vi "VI Server_Set Control Values from String Formats.vi"(6 "Options":T1, 8 "error in (no error)":errorcluster, 9 "Values":string[](array[string]), 10 "Labels":string[](array[string]), 11 "VI Server Cluster":T2={"Labels"=["Label", "Size", "Font", "Heght", "Width", "Ledding Denominator", "Ledding Nominator", "Label Number", "Microstep Resolution", "X", "Y", "Z", "Italic?", "Underlined?"], "Refs"=[], "VI Ref"=refnum}) -> (0 "error out":errorcluster, 3 "VI Server Cluster.DUP":T2={"Labels"=["Label", "Size", "Font", "Heght", "Width", "Ledding Denominator", "Ledding Nominator", "Label Number", "Microstep Resolution", "X", "Y", "Z", "Italic?", "Underlined?"], "Refs"=[], "VI Ref"=refnum}, 5 "FailedLabel":string)   [LabVIEW 2020, in "VI Server Toolkit LV2013.lvlib"]
doc: "<B>Set Control Values From String Formats.vi</B> and converts string values of the selected GUI objects onto original data type."
uses:
  VI Server Toolkit LV2013.lvlib
  VI Server_TypeDefs/VI Server_RefsCluster.ctl
  VI Server Libraries/VI Server Controls.llb/VI Server_GetSet Controls From String Format_Options.ctl
  <vilib>/userDefined/High Color/IMAQdx.ctl
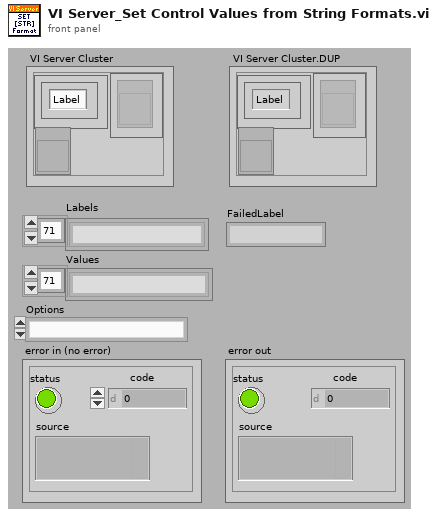
[diagram p1: front panel]
types:
  T1 = typedef "VI Server Toolkit LV2013.lvlib/VI Server_GetSet Controls From String Format_Options.ctl" = enum16{"", "If Ring Get Selection", "If Ring Set by Selection"}
  T2 = typedef "VI Server_RefsCluster.ctl" = cluster{"Labels":string[], "Refs":refnum<vi>[], "VI Ref":refnum<vi>}
  T3 = typedef "IMAQdx.ctl" = refnum<k21>
  T4 = typedef "LVStringsAndValuesArrayTypeDef_U32.ctl" = cluster{"String":string, "Value":u32}[]
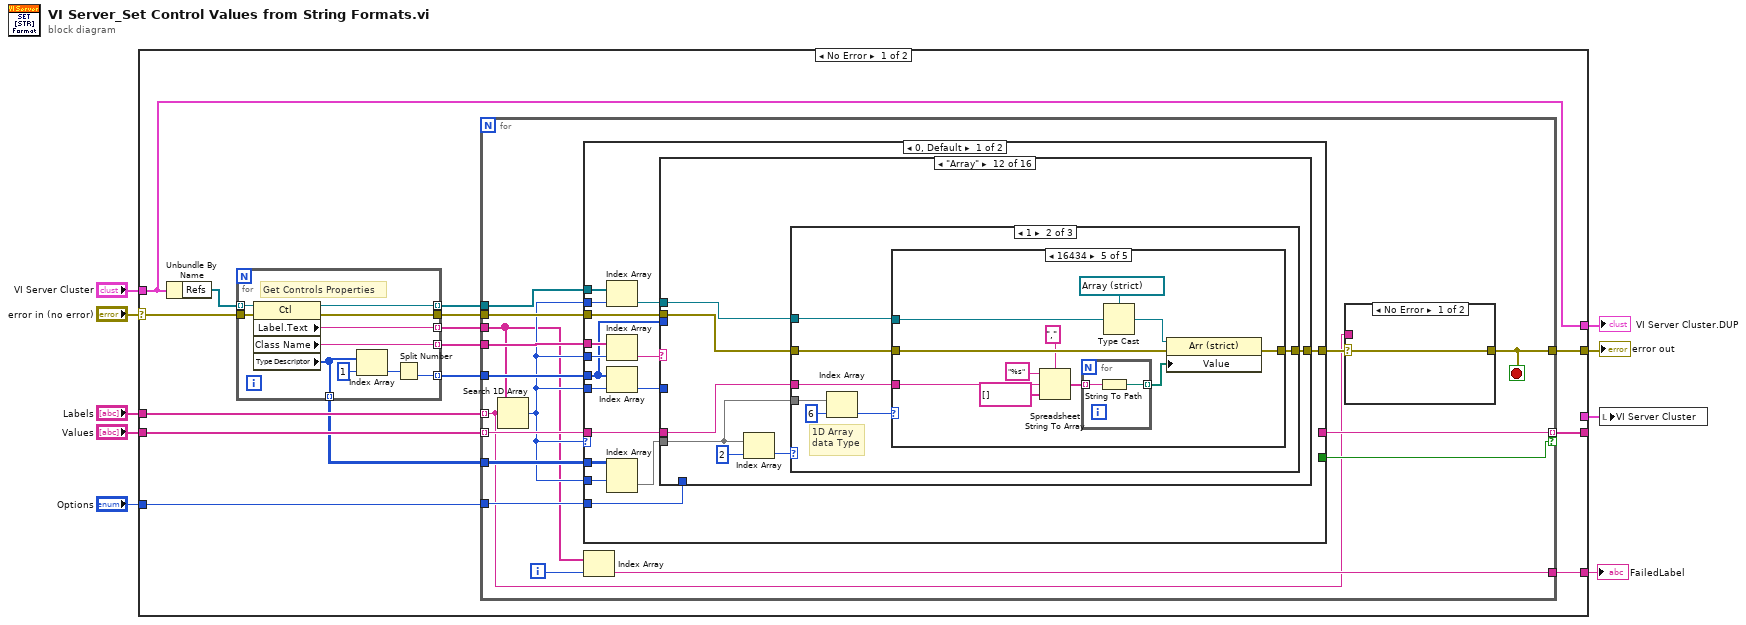
[diagram p0: block diagram]
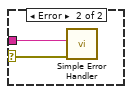
[diagram p2: hidden frame]
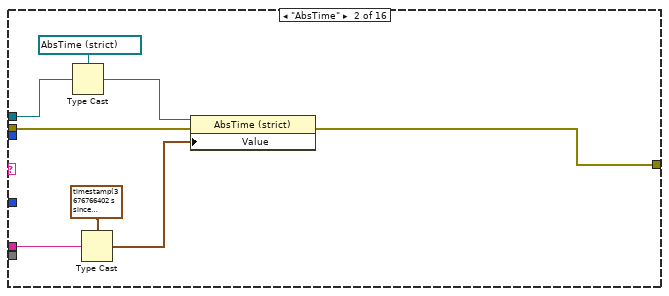
[diagram p4: hidden frame]
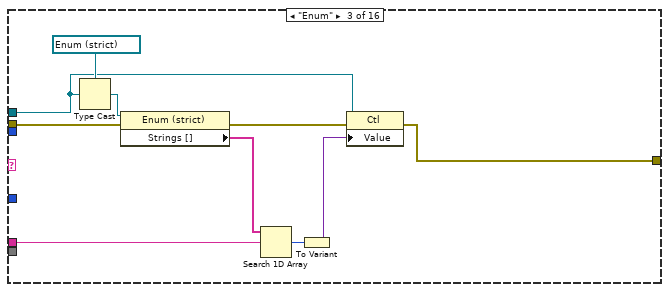
[diagram p5: hidden frame]
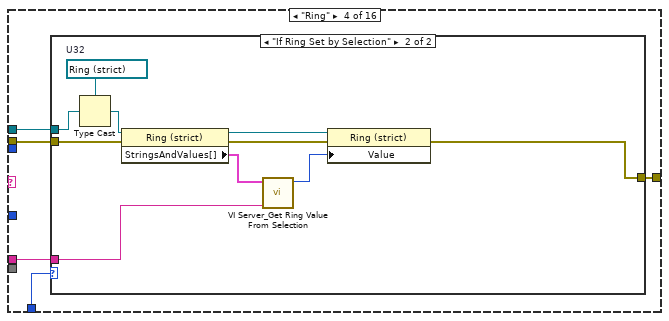
[diagram p6: hidden frame]
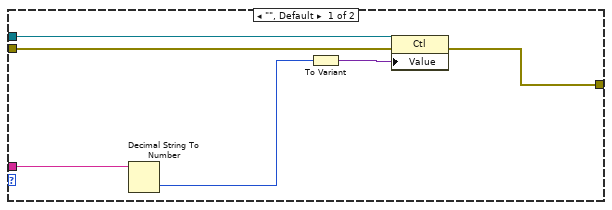
[diagram p7: hidden frame]
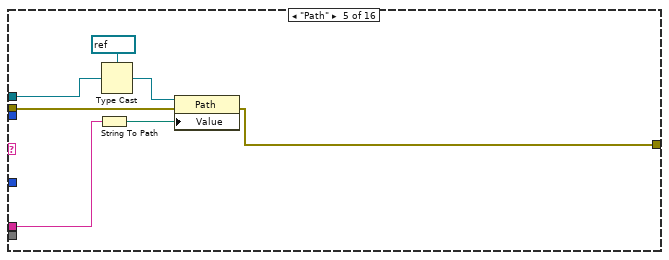
[diagram p8: hidden frame]
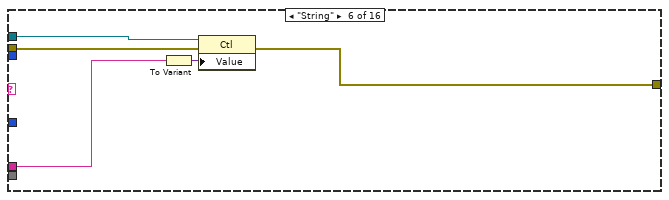
[diagram p9: hidden frame]
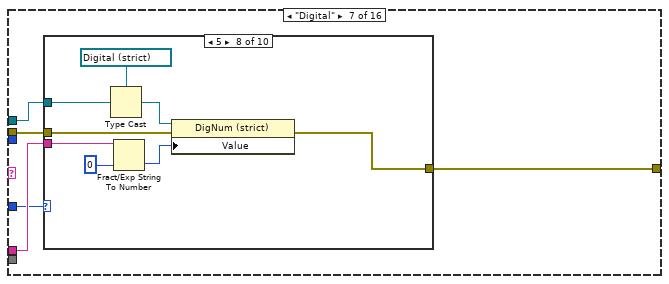
[diagram p10: hidden frame]
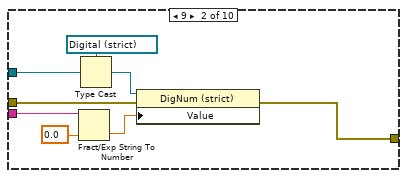
[diagram p12: hidden frame]
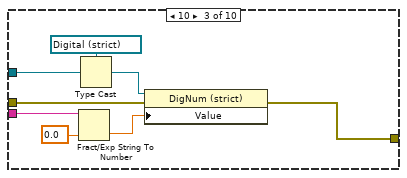
[diagram p13: hidden frame]
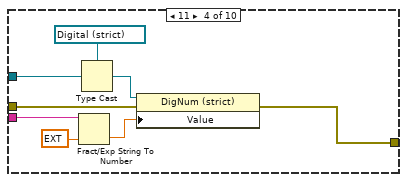
[diagram p14: hidden frame]
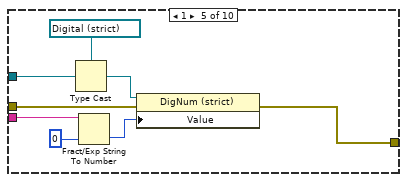
[diagram p15: hidden frame]
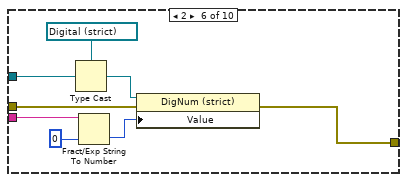
[diagram p16: hidden frame]
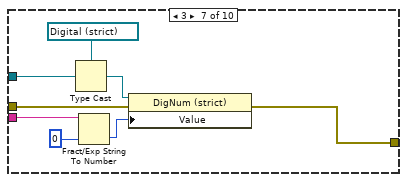
[diagram p17: hidden frame]
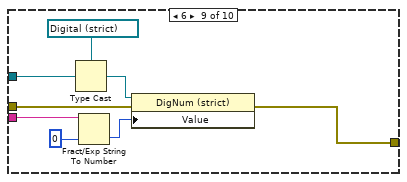
[diagram p18: hidden frame]
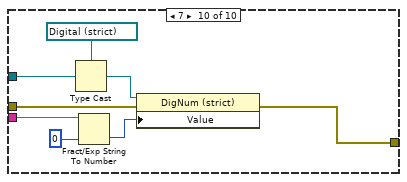
[diagram p19: hidden frame]
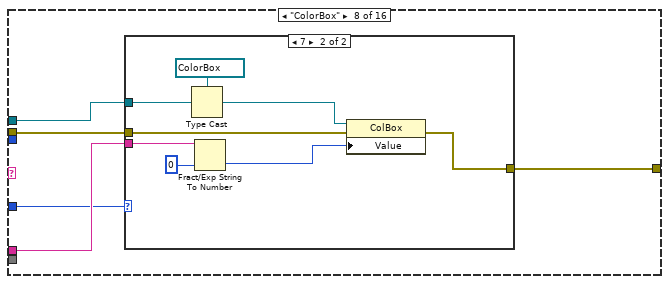
[diagram p20: hidden frame]
diagram:
  n1 = case shown="No Error" "error in (no error)" {
    selector: "error in (no error)" -> [w14 w655]
    tunnel: "Labels" -> [w19 _]
    tunnel: "Values" -> [w20 _]
    tunnel: [w13 w655] -> w7
    tunnel: [w12 _] -> w5
    tunnel: "VI Server Cluster" -> [w12 _]
    tunnel: "Options" -> [w15 _]
    tunnel: [_ w654] -> w2
    tunnel: [w11 _] -> _
    tunnel: [w10 _] -> w1
    frame No Error {
      n2 = Unbundle By Name(w12) -> ("Refs"=w18:refnum<vi>[])
      n3 = for {
        tunnel: w18 -> [w653] mode=indexing
        tunnel: w14 -> [w652]
        tunnel: [w651] -> w24 mode=indexing
        tunnel: [w650] -> w22 mode=indexing
        tunnel: [w649] -> w23 mode=indexing
        tunnel: [w648] -> w21
        tunnel: [w645] -> w17 mode=indexing
        tunnel: [w644] -> w16 mode=indexing
        # "Get Controls Properties"
        n4 = property class="Ctl"(reference=w653, error in=w652) -> (reference out=w649:refnum<vi>, error out=w648:errorcluster, "Label.Text"=w651:string, "Class Name"=w650:string, "Type Descriptor"=w644:i16[])
        n5 = Index Array(array=w644, index=1) -> (element=w646:i16)
        n6 = Split Number(x=w646) -> (lo(x)=w645:u8)  [unwired: 1 out]
      }
      n7 = for {
        tunnel: w19 -> [w25] mode=indexing
        tunnel: w24 -> [w30]
        tunnel: w23 -> [w38]
        tunnel: w22 -> [w40]
        tunnel: w20 -> [w39] mode=indexing
        tunnel: w21 -> [w37]
        tunnel: [w26] -> w13
        tunnel: w17 -> [w36]
        tunnel: w16 -> [w35]
        tunnel: w15 -> [w33]
        tunnel: [w32] -> w11 mode=indexing if=w31
        tunnel: [w28] -> w10
        i -> [w29]
        stop <- w26 stop-if-true
        n8 = Search 1D Array(1D array=w30, element=w25) -> (index of element=w34:i32)  [unwired: 1 out]
        n9 = case shown="0, Default" w34 {
          tunnel: w38 -> [w59 _]
          tunnel: w34 -> [w58 _]
          tunnel: w40 -> [w57 _]
          tunnel: w34 -> [w56 _]
          tunnel: w39 -> [w53 w642]
          tunnel: w37 -> [w52 w643]
          tunnel: [w51 w643] -> w27
          tunnel: w36 -> [w48 _]
          tunnel: w34 -> [w50 _]
          tunnel: w35 -> [w46 _]
          tunnel: w34 -> [w47 _]
          tunnel: w33 -> [w44 _]
          tunnel: [_ w642] -> w32
          tunnel: [_ TRUE] -> w31
          frame 0, Default {
            n10 = Index Array(array=w59, index=w58) -> (element=w54:refnum<vi>)
            n11 = Index Array(array=w57, index=w56) -> (element=w55:string)
            n12 = Index Array(array=w48, index=w50) -> (element=w49:u8)
            n13 = Index Array(array=w46, index (row)=w47) -> (element=w45:i16[])  [unwired: 1 in]
            n14 = case shown="\"Array\"" w55 {
              tunnel: w54 -> [_ w68 w71 w80 w102 w111 w114 w192 w206 w296 w303 w310 w492 w515 w546 w552]
              tunnel: w53 -> [_ w66 w76 w83 w105 w109 w113 w191 w205 w289 w301 w309 w490 w516 w547 w553]
              tunnel: w52 -> [w60 w64 w74 w82 w103 w108 w116 w194 w208 w298 w304 w314 w494 w517 w541 w554]
              tunnel: [w60 w63 w72 w81 w104 w107 w115 w193 w207 w297 w299 w313 w493 w514 w544 w551] -> w51
              tunnel: w49 -> [_ _ _ _ _ _ w112 w190 w204 _ _ _ w491 w513 _ _]
              tunnel: w48 -> [_ _ _ _ _ _ _ _ _ _ _ _ _ _ _ _]
              tunnel: w45 -> [_ _ _ _ _ _ _ _ _ _ _ w312 _ _ _ w550]
              tunnel: w44 -> [_ _ _ w79 _ _ _ _ _ _ _ _ _ _ _ _]
              frame "", Default {
              }
              frame "AbsTime" {
                n15 = Type Cast(type=refnum<vi> refnum ("UtilizationData.From"), x=w68) -> (*(type *) &x=w62:refnum<vi>)
                n16 = Type Cast(type=timestamp(3676766402.6552744 s since 1904-01-01) ("UtilizationData.From"), x=w66) -> (*(type *) &x=w61:timestamp)
                n17 = property class="AbsTime (strict)"(reference=w62, error in=w64, "Value"=w61) -> (error out=w63:errorcluster)  [unwired: 1 out]
              }
              frame "Enum" {
                n18 = Type Cast(type=refnum<vi> refnum ("Enum"), x=w71) -> (*(type *) &x=w77:refnum<vi>)
                n19 = property class="Enum (strict)"(reference=w77, error in=w74) -> (error out=w73:errorcluster, "Strings []"=w75:string[])  [unwired: 1 out]
                n20 = Search 1D Array(1D array=w75, element=w76) -> (index of element=w70:i32)  [unwired: 1 out]
                n21 = To Variant(anything=w70) -> (Variant=w69:variant)
                n22 = property class="Ctl"(reference=w71, error in=w73, "Value"=w69) -> (error out=w72:errorcluster)  [unwired: 1 out]
              }
              frame "Ring" {
                n23 = case shown="\"If Ring Set by Selection\"" w79 {
                  tunnel: w83 -> [w87 w93]
                  tunnel: w82 -> [w89 w98]
                  tunnel: [w88 w96] -> w81
                  tunnel: w80 -> [w85 w95]
                  frame "", Default {
                    n24 = Decimal String To Number(string=w87) -> (number=w86:i32)  [unwired: 2 in, 1 out]
                    n25 = To Variant(anything=w86) -> (Variant=w84:variant)
                    n26 = property class="Ctl"(reference=w85, error in=w89, "Value"=w84) -> (error out=w88:errorcluster)  [unwired: 1 out]
                  }
                  frame "If Ring Set by Selection" {
                    w90 = refnum<vi> refnum  # U32
                    n27 = Type Cast(type=w90, x=w95) -> (*(type *) &x=w99:refnum<vi>)
                    n28 = property class="Ring (strict)"(reference=w99, error in=w98) -> (reference out=w92:refnum<vi>, error out=w97:errorcluster, "StringsAndValues[]"=w94:T4)
                    n29 = call "VI Server_Get Ring Value From Selection.vi"("Item.Selected"=w93, "StringsAndValues[]"=w94) -> ("Value"=w91:u32)  [unwired: 9 in]
                    n30 = property class="Ring (strict)"(reference=w92, error in=w97, "Value"=w91) -> (error out=w96:errorcluster)  [unwired: 1 out]
                  }
                }
              }
              frame "Path" {
                n31 = String To Path(string=w105) -> (path=w106:path)
                n32 = Type Cast(type=refnum<vi> refnum ("Path"), x=w102) -> (*(type *) &x=w101:refnum<vi>)
                n33 = property class="Path"(reference=w101, error in=w103, "Value"=w106) -> (error out=w104:errorcluster)  [unwired: 1 out]
              }
              frame "String" {
                n34 = To Variant(anything=w109) -> (Variant=w110:variant)
                n35 = property class="Ctl"(reference=w111, error in=w108, "Value"=w110) -> (error out=w107:errorcluster)  [unwired: 1 out]
              }
              frame "Digital" {
                n36 = case shown="5" w112 {
                  tunnel: w116 -> [w117 w125 w133 w141 w149 w157 w165 w173 w181 w189]
                  tunnel: [w117 w124 w132 w140 w148 w156 w164 w172 w180 w188] -> w115
                  tunnel: w114 -> [_ w123 w131 w139 w147 w155 w163 w171 w179 w187]
                  tunnel: w113 -> [_ w121 w128 w137 w145 w153 w161 w169 w177 w185]
                  frame 0, Default {
                  }
                  frame 9 {
                    n37 = Fract/Exp String To Number(string=w121, default (0 dbl)=sgl 0.0) -> (number=w120:sgl)  [unwired: 3 out]
                    n38 = Type Cast(type=refnum<vi> refnum ("SGL"), x=w123) -> (*(type *) &x=w122:refnum<vi>)
                    n39 = property class="DigNum (strict)"(reference=w122, error in=w125, "Value"=w120) -> (error out=w124:errorcluster)  [unwired: 1 out]
                  }
                  frame 10 {
                    n40 = Fract/Exp String To Number(string=w128, default (0 dbl)=0.0) -> (number=w127:dbl)  [unwired: 3 out]
                    n41 = Type Cast(type=refnum<vi> refnum ("DBL"), x=w131) -> (*(type *) &x=w129:refnum<vi>)
                    n42 = property class="DigNum (strict)"(reference=w129, error in=w133, "Value"=w127) -> (error out=w132:errorcluster)  [unwired: 1 out]
                  }
                  frame 11 {
                    n43 = Fract/Exp String To Number(string=w137, default (0 dbl)=ext 0.0) -> (number=w136:ext)  [unwired: 3 out]
                    n44 = Type Cast(type=refnum<vi> refnum ("EXT"), x=w139) -> (*(type *) &x=w138:refnum<vi>)
                    n45 = property class="DigNum (strict)"(reference=w138, error in=w141, "Value"=w136) -> (error out=w140:errorcluster)  [unwired: 1 out]
                  }
                  frame 1 {
                    n46 = Type Cast(type=refnum<vi> refnum ("I8"), x=w147) -> (*(type *) &x=w146:refnum<vi>)
                    n47 = Fract/Exp String To Number(string=w145, default (0 dbl)=i8 0) -> (number=w144:i8)  [unwired: 3 out]
                    n48 = property class="DigNum (strict)"(reference=w146, error in=w149, "Value"=w144) -> (error out=w148:errorcluster)  [unwired: 1 out]
                  }
                  frame 2 {
                    n49 = Type Cast(type=refnum<vi> refnum ("I16"), x=w155) -> (*(type *) &x=w154:refnum<vi>)
                    n50 = Fract/Exp String To Number(string=w153, default (0 dbl)=i16 0) -> (number=w152:i16)  [unwired: 3 out]
                    n51 = property class="DigNum (strict)"(reference=w154, error in=w157, "Value"=w152) -> (error out=w156:errorcluster)  [unwired: 1 out]
                  }
                  frame 3 {
                    n52 = Type Cast(type=refnum<vi> refnum ("I32"), x=w163) -> (*(type *) &x=w162:refnum<vi>)
                    n53 = Fract/Exp String To Number(string=w161, default (0 dbl)=0) -> (number=w160:i32)  [unwired: 3 out]
                    n54 = property class="DigNum (strict)"(reference=w162, error in=w165, "Value"=w160) -> (error out=w164:errorcluster)  [unwired: 1 out]
                  }
                  frame 5 {
                    n55 = Type Cast(type=refnum<vi> refnum ("U8"), x=w171) -> (*(type *) &x=w170:refnum<vi>)
                    n56 = Fract/Exp String To Number(string=w169, default (0 dbl)=u8 0) -> (number=w168:u8)  [unwired: 3 out]
                    n57 = property class="DigNum (strict)"(reference=w170, error in=w173, "Value"=w168) -> (error out=w172:errorcluster)  [unwired: 1 out]
                  }
                  frame 6 {
                    n58 = Type Cast(type=refnum<vi> refnum ("U16"), x=w179) -> (*(type *) &x=w178:refnum<vi>)
                    n59 = Fract/Exp String To Number(string=w177, default (0 dbl)=u16 0) -> (number=w176:u16)  [unwired: 3 out]
                    n60 = property class="DigNum (strict)"(reference=w178, error in=w181, "Value"=w176) -> (error out=w180:errorcluster)  [unwired: 1 out]
                  }
                  frame 7 {
                    n61 = Type Cast(type=refnum<vi> refnum ("U32"), x=w187) -> (*(type *) &x=w186:refnum<vi>)
                    n62 = Fract/Exp String To Number(string=w185, default (0 dbl)=u32 0) -> (number=w184:u32)  [unwired: 3 out]
                    n63 = property class="DigNum (strict)"(reference=w186, error in=w189, "Value"=w184) -> (error out=w188:errorcluster)  [unwired: 1 out]
                  }
                }
              }
              frame "ColorBox" {
                n64 = case shown="7" w190 {
                  tunnel: w194 -> [w195 w203]
                  tunnel: [w195 w202] -> w193
                  tunnel: w192 -> [_ w201]
                  tunnel: w191 -> [_ w199]
                  frame 0, Default {
                  }
                  frame 7 {
                    n65 = Type Cast(type=refnum<vi> refnum ("Limits.RPM.Scale.Color<=1000"), x=w201) -> (*(type *) &x=w200:refnum<vi>)
                    n66 = Fract/Exp String To Number(string=w199, default (0 dbl)=u32 0) -> (number=w198:u32)  [unwired: 3 out]
                    n67 = property class="ColBox"(reference=w200, error in=w203, "Value"=w198) -> (error out=w202:errorcluster)  [unwired: 1 out]
                  }
                }
              }
              frame "Slide" {
                n68 = case shown="7" w204 {
                  tunnel: w208 -> [w209 w217 w226 w235 w243 w251 w259 w267 w275 w283]
                  tunnel: [w209 w216 w225 w234 w242 w250 w258 w266 w274 w282] -> w207
                  tunnel: w206 -> [_ w215 w224 w233 w241 w249 w257 w265 w273 w281]
                  tunnel: w205 -> [_ w213 w221 w231 w239 w247 w255 w263 w271 w279]
                  frame 0, Default {
                  }
                  frame 9 {
                    n69 = Fract/Exp String To Number(string=w213, default (0 dbl)=sgl 0.0) -> (number=w212:sgl)  [unwired: 3 out]
                    n70 = Type Cast(type=refnum<vi> refnum ("SGL 2"), x=w215) -> (*(type *) &x=w214:refnum<vi>)
                    n71 = property class="DigNum (strict)"(reference=w214, error in=w217, "Value"=w212) -> (reference out=w218:refnum<vi>, error out=w216:errorcluster)
                    n72 = Close Reference(reference=w218) -> ()  [unwired: 1 in, 1 out]
                  }
                  frame 10 {
                    n73 = Fract/Exp String To Number(string=w221, default (0 dbl)=0.0) -> (number=w220:dbl)  [unwired: 3 out]
                    n74 = Type Cast(type=refnum<vi> refnum ("DBL 2"), x=w224) -> (*(type *) &x=w222:refnum<vi>)
                    n75 = property class="DigNum (strict)"(reference=w222, error in=w226, "Value"=w220) -> (reference out=w227:refnum<vi>, error out=w225:errorcluster)
                    n76 = Close Reference(reference=w227) -> ()  [unwired: 1 in, 1 out]
                  }
                  frame 11 {
                    n77 = Fract/Exp String To Number(string=w231, default (0 dbl)=ext 0.0) -> (number=w230:ext)  [unwired: 3 out]
                    n78 = Type Cast(type=refnum<vi> refnum ("EXT 2"), x=w233) -> (*(type *) &x=w232:refnum<vi>)
                    n79 = property class="DigNum (strict)"(reference=w232, error in=w235, "Value"=w230) -> (error out=w234:errorcluster)  [unwired: 1 out]
                  }
                  frame 1 {
                    n80 = Type Cast(type=refnum<vi> refnum ("I8 2"), x=w241) -> (*(type *) &x=w240:refnum<vi>)
                    n81 = Fract/Exp String To Number(string=w239, default (0 dbl)=i8 0) -> (number=w238:i8)  [unwired: 3 out]
                    n82 = property class="DigNum (strict)"(reference=w240, error in=w243, "Value"=w238) -> (error out=w242:errorcluster)  [unwired: 1 out]
                  }
                  frame 2 {
                    n83 = Type Cast(type=refnum<vi> refnum ("I16 2"), x=w249) -> (*(type *) &x=w248:refnum<vi>)
                    n84 = Fract/Exp String To Number(string=w247, default (0 dbl)=i16 0) -> (number=w246:i16)  [unwired: 3 out]
                    n85 = property class="DigNum (strict)"(reference=w248, error in=w251, "Value"=w246) -> (error out=w250:errorcluster)  [unwired: 1 out]
                  }
                  frame 3 {
                    n86 = Type Cast(type=refnum<vi> refnum ("I32 2"), x=w257) -> (*(type *) &x=w256:refnum<vi>)
                    n87 = Fract/Exp String To Number(string=w255, default (0 dbl)=0) -> (number=w254:i32)  [unwired: 3 out]
                    n88 = property class="DigNum (strict)"(reference=w256, error in=w259, "Value"=w254) -> (error out=w258:errorcluster)  [unwired: 1 out]
                  }
                  frame 5 {
                    n89 = Type Cast(type=refnum<vi> refnum ("U8 2"), x=w265) -> (*(type *) &x=w264:refnum<vi>)
                    n90 = Fract/Exp String To Number(string=w263, default (0 dbl)=u8 0) -> (number=w262:u8)  [unwired: 3 out]
                    n91 = property class="DigNum (strict)"(reference=w264, error in=w267, "Value"=w262) -> (error out=w266:errorcluster)  [unwired: 1 out]
                  }
                  frame 6 {
                    n92 = Type Cast(type=refnum<vi> refnum ("U16 2"), x=w273) -> (*(type *) &x=w272:refnum<vi>)
                    n93 = Fract/Exp String To Number(string=w271, default (0 dbl)=u16 0) -> (number=w270:u16)  [unwired: 3 out]
                    n94 = property class="DigNum (strict)"(reference=w272, error in=w275, "Value"=w270) -> (error out=w274:errorcluster)  [unwired: 1 out]
                  }
                  frame 7 {
                    n95 = Type Cast(type=refnum<vi> refnum ("U32 2"), x=w281) -> (*(type *) &x=w280:refnum<vi>)
                    n96 = Fract/Exp String To Number(string=w279, default (0 dbl)=u32 0) -> (number=w278:u32)  [unwired: 3 out]
                    n97 = property class="DigNum (strict)"(reference=w280, error in=w283, "Value"=w278) -> (error out=w282:errorcluster)  [unwired: 1 out]
                  }
                }
              }
              frame "Boolean" {
                n98 = Type Cast(type=refnum<vi> refnum ("Boolean"), x=w296) -> (*(type *) &x=w294:refnum<vi>)
                n99 = Equal?(x=w289, y="TRUE" ("x")) -> (x = y?=w292:bool)
                n100 = Equal?(x=w289, y="ON" ("x")) -> (x = y?=w288:bool)
                n101 = Equal?(x=w289, y="1" ("x")) -> (x = y?=w287:bool)
                n102 = Compound Arithmetic op=OR(w292, w288, w287) -> (w286:bool)
                n103 = Type Cast(type=FALSE ("Value"), x=w286) -> (*(type *) &x=w284:bool)
                n104 = property class="Bool (strict)"(reference=w294, error in=w298, "Value"=w284) -> (error out=w297:errorcluster)  [unwired: 1 out]
              }
              frame "Table" {
                n105 = Type Cast(type=refnum<vi> refnum ("Image Statistics Table"), x=w303) -> (*(type *) &x=w306:refnum<vi>)
                n106 = Spreadsheet String To Array(delimiter (Tab)=",", format string="%s", spreadsheet string=w301, array type (2D Dbl)=string[][] []) -> (array=w300:string[][])
                n107 = property class="Tbl (strict)"(reference=w306, error in=w304, "Value"=w300) -> (error out=w299:errorcluster)  [unwired: 1 out]
              }
              frame "Array" {
                n108 = Index Array(array=w312, index=2) -> (element=w311:i16)
                n109 = case shown="1" w311 {
                  tunnel: w312 -> [_ w322 w374]
                  tunnel: w314 -> [w316 w321 w373]
                  tunnel: [w316 w319 w372] -> w313
                  tunnel: w310 -> [_ w318 w371]
                  tunnel: w309 -> [_ w317 w370]
                  frame 0, Default {
                  }
                  frame 1 {
                    # "1D Array\ndata Type"
                    n110 = Index Array(array=w322, index=6) -> (element=w320:i16)
                    n111 = case shown="16434" w320 {
                      tunnel: w318 -> [_ w334 w344 w354 w365]
                      tunnel: [w324 w332 w342 w352 w363] -> w319
                      tunnel: w321 -> [w324 w331 w341 w351 w362]
                      tunnel: w317 -> [_ w327 w338 w347 w360]
                      frame 0, Default {
                      }
                      frame 16394 {
                        n112 = Spreadsheet String To Array(delimiter (Tab)=",", format string="%0.6f", spreadsheet string=w327, array type (2D Dbl)=dbl[] []) -> (array=w325:dbl[])
                        n113 = Type Cast(type=refnum<vi> refnum ("Array"), x=w334) -> (*(type *) &x=w333:refnum<vi>)
                        n114 = property class="Arr (strict)"(reference=w333, error in=w331, "Value"=w325) -> (error out=w332:errorcluster)  [unwired: 1 out]
                      }
                      frame 16389 {
                        n115 = Spreadsheet String To Array(delimiter (Tab)=",", format string="%d", spreadsheet string=w338, array type (2D Dbl)=u8[] []) -> (array=w336:u8[])
                        n116 = Type Cast(type=refnum<vi> refnum ("Message.Payload"), x=w344) -> (*(type *) &x=w343:refnum<vi>)
                        n117 = property class="Arr (strict)"(reference=w343, error in=w341, "Value"=w336) -> (error out=w342:errorcluster)  [unwired: 1 out]
                      }
                      frame 16432 {
                        n118 = Spreadsheet String To Array(delimiter (Tab)=",", format string="%s", spreadsheet string=w347, array type (2D Dbl)=string[] []) -> (array=w345:string[])
                        n119 = Type Cast(type=refnum<vi> refnum ("1D String"), x=w354) -> (*(type *) &x=w353:refnum<vi>)
                        n120 = property class="Arr (strict)"(reference=w353, error in=w351, "Value"=w345) -> (error out=w352:errorcluster)  [unwired: 1 out]
                      }
                      frame 16434 {
                        n121 = Spreadsheet String To Array(delimiter (Tab)=",", format string="%s", spreadsheet string=w360, array type (2D Dbl)=string[] []) -> (array=w356:string[])
                        n122 = for {
                          tunnel: w356 -> [w367] mode=indexing
                          tunnel: [w366] -> w355 mode=indexing
                          n123 = String To Path(string=w367) -> (path=w366:path)
                        }
                        n124 = Type Cast(type=refnum<vi> refnum ("Array"), x=w365) -> (*(type *) &x=w364:refnum<vi>)
                        n125 = property class="Arr (strict)"(reference=w364, error in=w362, "Value"=w355) -> (error out=w363:errorcluster)  [unwired: 1 out]
                      }
                    }
                  }
                  frame 2 {
                    n126 = Index Array(array=w374, index=8) -> (element=w369:i16)
                    n127 = Split Number(x=w369) -> (lo(x)=w368:u8)  [unwired: 1 out]
                    n128 = case shown="32" w368 {
                      tunnel: w371 -> [_ w386 w396 w406 w416 w426 w436 w446 w456 w466 w476 w487]
                      tunnel: [w376 w384 w394 w404 w414 w424 w434 w444 w454 w464 w474 w485] -> w372
                      tunnel: w373 -> [w376 w383 w393 w403 w413 w423 w433 w443 w453 w463 w473 w484]
                      tunnel: w370 -> [_ w380 w390 w400 w410 w420 w430 w440 w450 w460 w470 w483]
                      frame 0, Default {
                      }
                      frame 1 {
                        n129 = Spreadsheet String To Array(delimiter (Tab)=",", format string="%d", spreadsheet string=w380, array type (2D Dbl)=i8[][] []) -> (array=w378:i8[][])
                        n130 = Type Cast(type=refnum<vi> refnum ("Array"), x=w386) -> (*(type *) &x=w385:refnum<vi>)
                        n131 = property class="Arr (strict)"(reference=w385, error in=w383, "Value"=w378) -> (error out=w384:errorcluster)  [unwired: 1 out]
                      }
                      frame 2 {
                        n132 = Spreadsheet String To Array(delimiter (Tab)=",", format string="%d", spreadsheet string=w390, array type (2D Dbl)=i16[][] []) -> (array=w388:i16[][])
                        n133 = Type Cast(type=refnum<vi> refnum ("Array"), x=w396) -> (*(type *) &x=w395:refnum<vi>)
                        n134 = property class="Arr (strict)"(reference=w395, error in=w393, "Value"=w388) -> (error out=w394:errorcluster)  [unwired: 1 out]
                      }
                      frame 3 {
                        n135 = Spreadsheet String To Array(delimiter (Tab)=",", format string="%d", spreadsheet string=w400, array type (2D Dbl)=i32[][] []) -> (array=w398:i32[][])
                        n136 = Type Cast(type=refnum<vi> refnum ("Array"), x=w406) -> (*(type *) &x=w405:refnum<vi>)
                        n137 = property class="Arr (strict)"(reference=w405, error in=w403, "Value"=w398) -> (error out=w404:errorcluster)  [unwired: 1 out]
                      }
                      frame 5 {
                        n138 = Spreadsheet String To Array(delimiter (Tab)=",", format string="%d", spreadsheet string=w410, array type (2D Dbl)=u8[][] []) -> (array=w408:u8[][])
                        n139 = Type Cast(type=refnum<vi> refnum ("Array"), x=w416) -> (*(type *) &x=w415:refnum<vi>)
                        n140 = property class="Arr (strict)"(reference=w415, error in=w413, "Value"=w408) -> (error out=w414:errorcluster)  [unwired: 1 out]
                      }
                      frame 6 {
                        n141 = Spreadsheet String To Array(delimiter (Tab)=",", format string="%d", spreadsheet string=w420, array type (2D Dbl)=u16[][] []) -> (array=w418:u16[][])
                        n142 = Type Cast(type=refnum<vi> refnum ("Array"), x=w426) -> (*(type *) &x=w425:refnum<vi>)
                        n143 = property class="Arr (strict)"(reference=w425, error in=w423, "Value"=w418) -> (error out=w424:errorcluster)  [unwired: 1 out]
                      }
                      frame 7 {
                        n144 = Spreadsheet String To Array(delimiter (Tab)=",", format string="%d", spreadsheet string=w430, array type (2D Dbl)=u32[][] []) -> (array=w428:u32[][])
                        n145 = Type Cast(type=refnum<vi> refnum ("Array"), x=w436) -> (*(type *) &x=w435:refnum<vi>)
                        n146 = property class="Arr (strict)"(reference=w435, error in=w433, "Value"=w428) -> (error out=w434:errorcluster)  [unwired: 1 out]
                      }
                      frame 9 {
                        n147 = Spreadsheet String To Array(delimiter (Tab)=",", format string="%f", spreadsheet string=w440, array type (2D Dbl)=sgl[][] []) -> (array=w438:sgl[][])
                        n148 = Type Cast(type=refnum<vi> refnum ("Array"), x=w446) -> (*(type *) &x=w445:refnum<vi>)
                        n149 = property class="Arr (strict)"(reference=w445, error in=w443, "Value"=w438) -> (error out=w444:errorcluster)  [unwired: 1 out]
                      }
                      frame 10 {
                        n150 = Spreadsheet String To Array(delimiter (Tab)=",", format string="%f", spreadsheet string=w450, array type (2D Dbl)=dbl[][] []) -> (array=w448:dbl[][])
                        n151 = Type Cast(type=refnum<vi> refnum ("Array"), x=w456) -> (*(type *) &x=w455:refnum<vi>)
                        n152 = property class="Arr (strict)"(reference=w455, error in=w453, "Value"=w448) -> (error out=w454:errorcluster)  [unwired: 1 out]
                      }
                      frame 11 {
                        n153 = Spreadsheet String To Array(delimiter (Tab)=",", format string="%f", spreadsheet string=w460, array type (2D Dbl)=ext[][] []) -> (array=w458:ext[][])
                        n154 = Type Cast(type=refnum<vi> refnum ("Array"), x=w466) -> (*(type *) &x=w465:refnum<vi>)
                        n155 = property class="Arr (strict)"(reference=w465, error in=w463, "Value"=w458) -> (error out=w464:errorcluster)  [unwired: 1 out]
                      }
                      frame 48 {
                        n156 = Spreadsheet String To Array(delimiter (Tab)=",", format string="%s", spreadsheet string=w470, array type (2D Dbl)=string[][] []) -> (array=w468:string[][])
                        n157 = Type Cast(type=refnum<vi> refnum ("Array"), x=w476) -> (*(type *) &x=w475:refnum<vi>)
                        n158 = property class="Arr (strict)"(reference=w475, error in=w473, "Value"=w468) -> (error out=w474:errorcluster)  [unwired: 1 out]
                      }
                      frame 50 {
                        n159 = Spreadsheet String To Array(delimiter (Tab)=",", format string="%s", spreadsheet string=w483, array type (2D Dbl)=string[][] []) -> (array=w479:string[][])
                        n160 = for {
                          tunnel: w479 -> [w489] mode=indexing
                          tunnel: [w488] -> w478 mode=indexing
                          n161 = String To Path(string=w489) -> (path=w488:path[])
                        }
                        n162 = Type Cast(type=refnum<vi> refnum ("Array"), x=w487) -> (*(type *) &x=w486:refnum<vi>)
                        n163 = property class="Arr (strict)"(reference=w486, error in=w484, "Value"=w478) -> (error out=w485:errorcluster)  [unwired: 1 out]
                      }
                    }
                  }
                }
              }
              frame "MulticolumnListbox" {
                n164 = case shown="3" w491 {
                  tunnel: w494 -> [w495 w500 w511]
                  tunnel: [w495 w499 w510] -> w493
                  tunnel: w492 -> [_ w502 w512]
                  tunnel: w490 -> [_ w497 w507]
                  frame 0, Default {
                  }
                  frame 3 {
                    n165 = Decimal String To Number(string=w497) -> (number=w496:i32)  [unwired: 2 in, 1 out]
                    n166 = Type Cast(type=refnum<vi> refnum ("Controls Description"), x=w502) -> (*(type *) &x=w498:refnum<vi>)
                    n167 = property class="MCListbox (strict)"(reference=w498, error in=w500, "Value"=w496) -> (error out=w499:errorcluster)  [unwired: 1 out]
                  }
                  frame 64 {
                    n168 = Spreadsheet String To Array(delimiter (Tab)=",", format string="%s", spreadsheet string=w507, array type (2D Dbl)=i32[] [] ("Value")) -> (array=w503:i32[])
                    n169 = Type Cast(type=refnum<vi> refnum ("Controls Description"), x=w512) -> (*(type *) &x=w509:refnum<vi>)
                    n170 = property class="MCListbox (strict)"(reference=w509, error in=w511, "Value"=w503) -> (error out=w510:errorcluster)  [unwired: 1 out]
                  }
                }
              }
              frame "GenClassTagRef" {
                n171 = case shown="112" w513 {
                  tunnel: w517 -> [w518 w528 w538]
                  tunnel: w516 -> [_ w527 w537]
                  tunnel: w515 -> [_ w526 w536]
                  tunnel: [w518 w525 w535] -> w514
                  frame 0, Default {
                  }
                  frame 1 {
                    n172 = Type Cast(type=refnum<vi> refnum ("Camera.Left"), x=w526) -> (*(type *) &x=w522:refnum<vi>)
                    n173 = Unflatten From String(type=T3 refnum ("Camera.Ref"), binary string=w527, error in (no error)=w528) -> (value=w521:T3, error out=w523:errorcluster)  [unwired: 2 in, 1 out]
                    n174 = property class="IMAQdx (strict)"(reference=w522, error in=w523, "Value"=w521) -> (error out=w520:errorcluster)  [unwired: 1 out]
                    n175 = call <vilib>:"Simple Error Handler.vi"("error in (no error)"=w520) -> ()  [unwired: 4 in, 5 out]
                    n176 = call "Error 74_ClearEmptyFlattenedStringRecovery.vi"("error in"=w520) -> ("error out"=w525:errorcluster)  [unwired: 3 in, 1 out]
                  }
                  frame 112 {
                    n177 = Type Cast(type=refnum<vi> refnum ("Camera.Ref"), x=w536) -> (*(type *) &x=w533:refnum<vi>)
                    n178 = Unflatten From String(type=T3 refnum ("Camera.Ref"), binary string=w537, error in (no error)=w538) -> (value=w532:T3, error out=w534:errorcluster)  [unwired: 2 in, 1 out]
                    n179 = property class="IMAQdx (strict)"(reference=w533, error in=w534, "Value"=w532) -> (error out=w531:errorcluster)  [unwired: 1 out]
                    n180 = call <vilib>:"Simple Error Handler.vi"("error in (no error)"=w531) -> ()  [unwired: 4 in, 5 out]
                    n181 = call "Error 74_ClearEmptyFlattenedStringRecovery.vi"("error in"=w531) -> ("error out"=w535:errorcluster)  [unwired: 3 in, 1 out]
                  }
                }
              }
              frame "VISAResourceName" {
                n182 = call <vilib>:"Trim Whitespace.vi"("string"=w547) -> ("trimmed string"=w540:string)  [unwired: 1 in]
                n183 = Type Cast(type=refnum<vi> refnum ("VISA resource name"), x=w546) -> (*(type *) &x=w545:refnum<vi>)
                n184 = Type Cast(type=refnum<visa-resource-name> refnum ("GPS.VISA.ResourceName"), x=w540) -> (*(type *) &x=w539:refnum<visa-resource-name>)
                n185 = property class="VISAName"(reference=w545, error in=w541, "Value"=w539) -> (error out=w544:errorcluster)  [unwired: 1 out]
              }
              frame "DAQmxName" {
                n186 = Index Array(array=w550) -> (element=w549:i16)  [unwired: 1 in]
                n187 = call <vilib>:"Trim Whitespace.vi"("string"=w553) -> ("trimmed string"=w548:string)  [unwired: 1 in]
                n188 = case shown="18, 22, 28, 30" w549 {
                  tunnel: w554 -> [w555 w559 w569 w577 w586 w595 w601 w613 w620 w625 w635]
                  tunnel: w548 -> [_ w557 w568 w576 w584 w593 w603 w612 w619 w628 w637]
                  tunnel: w552 -> [_ w564 w573 w582 w591 w600 w608 w616 w624 w632 w640]
                  tunnel: [w555 w560 w570 w578 w588 w597 w607 w615 w623 w630 w639] -> w551
                  frame 0, Default {
                  }
                  frame 26, 38 {
                    n189 = Type Cast(type=refnum<vi> refnum ("CamTriggerGenerator.Counter"), x=w564) -> (*(type *) &x=w563:refnum<vi>)
                    n190 = Type Cast(type=tag "" ("CamTriggerGenerator.Counter"), x=w557) -> (*(type *) &x=w556:tag)
                    n191 = property class="DAQmxName"(reference=w563, error in=w559, "Value"=w556) -> (error out=w561:errorcluster)  [unwired: 1 out]
                    n192 = call "Error 74_ClearEmptyFlattenedStringRecovery.vi"("error in"=w561) -> ("error out"=w560:errorcluster)  [unwired: 3 in, 1 out]
                  }
                  frame 24 {
                    n193 = Type Cast(type=refnum<vi> refnum ("DAQmx.Device"), x=w573) -> (*(type *) &x=w572:refnum<vi>)
                    n194 = Type Cast(type=tag "" ("DAQmx.Device"), x=w568) -> (*(type *) &x=w567:tag)
                    n195 = property class="DAQmxName"(reference=w572, error in=w569, "Value"=w567) -> (error out=w571:errorcluster)  [unwired: 1 out]
                    n196 = call "Error 74_ClearEmptyFlattenedStringRecovery.vi"("error in"=w571) -> ("error out"=w570:errorcluster)  [unwired: 3 in, 1 out]
                  }
                  frame 18, 22, 28, 30 {
                    n197 = Type Cast(type=refnum<vi> refnum ("CamTriggerGenerator.Counter"), x=w582) -> (*(type *) &x=w581:refnum<vi>)
                    n198 = Type Cast(type=tag "Dev2/port1/line3" ("DAQ.GPM.DigitalLine"), x=w576) -> (*(type *) &x=w575:tag)
                    n199 = property class="DAQmxName"(reference=w581, error in=w577, "Value"=w575) -> (error out=w579:errorcluster)  [unwired: 1 out]
                    n200 = call "Error 74_ClearEmptyFlattenedStringRecovery.vi"("error in"=w579) -> ("error out"=w578:errorcluster)  [unwired: 3 in, 1 out]
                  }
                  frame 32 {
                    n201 = Type Cast(type=refnum<vi> refnum ("DAQmx.Digital Output"), x=w591) -> (*(type *) &x=w590:refnum<vi>)
                    n202 = Type Cast(type=tag "" ("DAQmx.Digital Output"), x=w584) -> (*(type *) &x=w585:tag)
                    n203 = property class="DAQmxName"(reference=w590, error in=w586, "Value"=w585) -> (error out=w589:errorcluster)  [unwired: 1 out]
                    n204 = call "Error 74_ClearEmptyFlattenedStringRecovery.vi"("error in"=w589) -> ("error out"=w588:errorcluster)  [unwired: 3 in, 1 out]
                  }
                  frame 34 {
                    n205 = Type Cast(type=refnum<vi> refnum ("DAQmx.Digital Output"), x=w600) -> (*(type *) &x=w599:refnum<vi>)
                    n206 = Type Cast(type=tag "Dev2/ai1" ("DAQ.EngineTilt.Channel"), x=w593) -> (*(type *) &x=w594:tag)
                    n207 = property class="DAQmxName"(reference=w599, error in=w595, "Value"=w594) -> (error out=w598:errorcluster)  [unwired: 1 out]
                    n208 = call "Error 74_ClearEmptyFlattenedStringRecovery.vi"("error in"=w598) -> ("error out"=w597:errorcluster)  [unwired: 3 in, 1 out]
                  }
                  frame 40 {
                    n209 = Type Cast(type=refnum<vi> refnum ("IlluminationControl.DigitalLines"), x=w608) -> (*(type *) &x=w606:refnum<vi>)
                    n210 = Type Cast(type=tag "Dev1/ctr0" ("Engine.FuelPump.DAQmx.Counter"), x=w603) -> (*(type *) &x=w602:tag)
                    n211 = property class="DAQmxName"(reference=w606, error in=w601, "Value"=w602) -> (error out=w607:errorcluster)  [unwired: 1 out]
                  }
                  frame 42, 48 {
                    n212 = Type Cast(type=refnum<vi> refnum ("Engine.FuelPump.PauseTrigger.DO"), x=w616) -> (*(type *) &x=w614:refnum<vi>)
                    n213 = Type Cast(type=tag "Dev1/port0/line7" ("Engine.FuelPump.PauseTrigger.DO"), x=w612) -> (*(type *) &x=w610:tag)
                    n214 = property class="DAQmxName"(reference=w614, error in=w613, "Value"=w610) -> (error out=w615:errorcluster)  [unwired: 1 out]
                  }
                  frame 44 {
                    n215 = Type Cast(type=refnum<vi> refnum ("IlluminationControl.DigitalLines"), x=w624) -> (*(type *) &x=w622:refnum<vi>)
                    n216 = Type Cast(type=tag "Dev2/port0/line0:1" ("IlluminationControl.DigitalLines"), x=w619) -> (*(type *) &x=w618:tag)
                    n217 = property class="DAQmxName"(reference=w622, error in=w620, "Value"=w618) -> (error out=w623:errorcluster)  [unwired: 1 out]
                  }
                  frame 36, 46 {
                    n218 = Type Cast(type=refnum<vi> refnum ("Engine.FuelPump.PauseTriggerSource"), x=w632) -> (*(type *) &x=w631:refnum<vi>)
                    n219 = Type Cast(type=tag "Output Terminal" ("CamTriggerGenerator.OutputTerminal"), x=w628) -> (*(type *) &x=w626:tag)
                    n220 = property class="DAQmxName"(reference=w631, error in=w625, "Value"=w626) -> (error out=w630:errorcluster)  [unwired: 1 out]
                  }
                  frame 50 {
                    n221 = Type Cast(type=refnum<vi> refnum ("DAQmx.RPM.FrequencyMonitor.DigitalLine"), x=w640) -> (*(type *) &x=w638:refnum<vi>)
                    n222 = Type Cast(type=tag "" ("DAQmx.RPM.FrequencyMonitor.DigitalLine"), x=w637) -> (*(type *) &x=w636:tag)
                    n223 = property class="DAQmxName"(reference=w638, error in=w635, "Value"=w636) -> (error out=w639:errorcluster)  [unwired: 1 out]
                  }
                }
              }
            }
          }
          frame -1 {
          }
        }
        n224 = Index Array(array=w30, index=w29) -> (element=w28:string)
        n225 = case shown="No Error" w27 {
          selector: w27 -> [w41 w43]
          tunnel: [w41 _] -> w26
          tunnel: w25 -> [_ w42]
          frame No Error {
          }
          frame Error {
            n226 = call <vilib>:"Simple Error Handler.vi"("error source (\" \")"=w42, "error in (no error)"=w43) -> ()  [unwired: 3 in, 5 out]
          }
        }
      }
    }
    frame Error {
      n227 = call "VI Server_Empty VI Server Cluster.vi"() -> ("VI Server Cluster"=w654:T2)  [unwired: 7 in]
    }
  }
  "error out" <- w7
  "VI Server Cluster.DUP" <- w5
  "FailedLabel" <- w1
  n228 = local write "VI Server Cluster"(w2) -> ()
